vi "Append 1D Column Double.vi"(6 "Font":refnum<class "Style.lvclass">, 8 "error in (no error)":errorcluster, 10 "Value":dbl[](array[numeric]), 11 "MS-Excel in":refnum<class "MS-Excel.lvclass">) -> (0 "error out":errorcluster, 3 "MS-Excel out":refnum<class "MS-Excel.lvclass">)   [LabVIEW 2017, in "LabVIEW NPOI.lvlib" / "MS-Excel.lvclass"]
doc: "Appends column-wise the wire <b>Value</b> as 1D array of doubles to the associated workbook to the <b>Document</b>."
uses:
  MS-Excel.lvclass
  Styles/Style/Style.lvclass
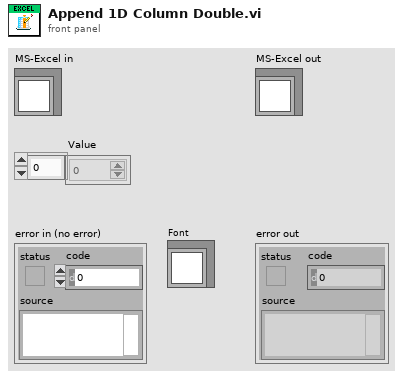
[diagram p1: front panel]
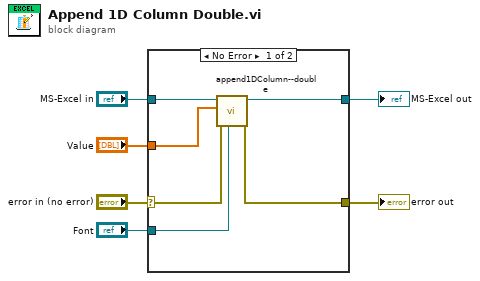
[diagram p0: block diagram]
diagram:
  n1 = case shown="No Error" "error in (no error)" {
    selector: "error in (no error)" -> [w9 w14]
    tunnel: [w8 w14] -> w5
    tunnel: [w11 w13] -> w3
    tunnel: "MS-Excel in" -> [w12 w13]
    tunnel: "Value" -> [w10 _]
    tunnel: "Font" -> [w7 _]
    frame No Error {
      n2 = call-dynamic "append1DColumn--double.vi"("Style"=w7, "error in (no error)"=w9, "Value"=w10, "MS-Excel in"=w12) -> ("error out"=w8:errorcluster, "MS-Excel out"=w11:refnum<class "MS-Excel.lvclass">)  [unwired: 6 in]
    }
    frame Error {
    }
  }
  "error out" <- w5
  "MS-Excel out" <- w3
